vi "motor_event.vi"() -> ()   [LabVIEW 2013]
panel:
  out "motor event":refnum<user-event>
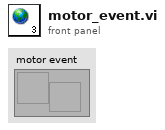
[diagram p1: front panel]
diagram:
